vi "Calc - dPAMB.vi"(11 "00-00-9220":dbl[](array[numeric])) -> (3 "dPAMB":dbl)   [LabVIEW 2018, in "Controller (Host).lvlib"]
uses:
  Controller (Host).lvlib
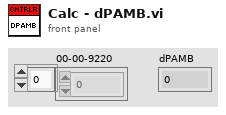
[diagram p1: front panel]
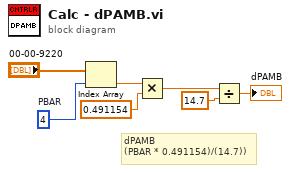
[diagram p0: block diagram]
diagram:
  w7 = 4  # PBAR
  # "dPAMB\n(PBAR * 0.491154)/(14.7))"
  n1 = Index Array(array="00-00-9220", index=w7) -> (element=w1:dbl)
  n2 = Multiply(x=w1, y=0.491154) -> (x*y=w3:dbl)
  n3 = Divide(x=w3, y=14.7 ("x")) -> (x/y=→"dPAMB":dbl)
